vi "Create Temporary File.vi"(8 "Error In":errorcluster, 11 "SFTP In":refnum<class "SFTP.lvclass">) -> (0 "Error Out":errorcluster, 1 "Remote Link Path":string, 2 "Remote Source Path":string, 3 "SFTP Out":refnum<class "SFTP.lvclass">)   [LabVIEW 2018, in "Tests.lvlib" / "SFTP.lvlib"]
uses:
  SFTP.lvlib
  src/Toolkit/API/SFTP/SFTP.lvclass
  src/Toolkit/API/SFTP File/API/Typedefs/Flags.ctl
  src/Toolkit/API/SFTP File/SFTP File.lvclass
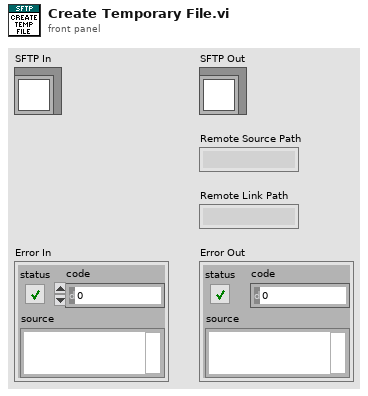
[diagram p1: front panel]
types:
  T1 = typedef "Toolkit.lvlib/SFTP File.lvclass/Flags.ctl" = cluster{"Read":bool, "Write":bool, "Append":bool, "Create":bool, "Truncate":bool, "Exclude":bool}
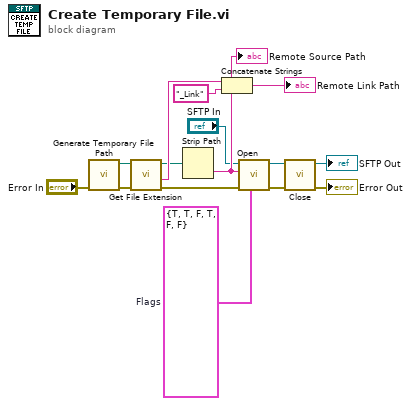
[diagram p0: block diagram]
diagram:
  w1 = T1 {"Read"=TRUE, "Write"=TRUE, "Append"=FALSE, "Create"=TRUE, "Truncate"=FALSE, "Exclude"=FALSE}  # Flags
  n1 = call <vilib>:"Generate Temporary File Path.vi"("error in (no error)"="Error In") -> ("error out"=w10:errorcluster, "Unique Temporary File Path"=w8:path)  [unwired: 9 in]
  n2 = call <vilib>:"Get File Extension.vi"("error in (no error)"=w10, "file"=w8) -> ("error out"=w11:errorcluster, "filename without extension"=w12:string, "dup file"=w9:path)  [unwired: 5 in, 2 out]
  n3 = Strip Path(path=w9) -> (name=w14:string)  [unwired: 1 out]
  "Remote Source Path" <- w14
  n4 = Concatenate Strings(w12, "_Link" ("string")) -> (→"Remote Link Path":string)
  n5 = call "Open.vi"("Flags"=w1, "Error In"=w11, "Remote Path"=w14, "SFTP"="SFTP In") -> ("Error Out"=w3:errorcluster, "SFTP File"=w2:refnum<class "SFTP File.lvclass">)  [unwired: 6 in]
  n6 = call "Close.vi"("Error In"=w3, "SFTP File"=w2) -> ("Error Out"=→"Error Out":errorcluster, "SFTP"=→"SFTP Out":refnum<class "SFTP.lvclass">)  [unwired: 8 in]
